vi "Exercise9.2-Basic Sine RX.vi"() -> ()   [LabVIEW 2013]
uses:
  <instrlib>/niUSRP/niUSRP Fetch Rx Data (CDB WDT).vi
  <vilib>/express/express analysis/Spectral/Block/exnSpectralBlock spectral measurements RMS poly.vi
  <vilib>/express/express analysis/Spectral/Block/exnSpectralBlock spectral measurements RMS WFM.vi
  <vilib>/express/express analysis/Spectral/XNode/ExpressSpectralMeasurementsBlockNode.xnode
panel:
  out "Spectrum":cluster{"f0":dbl, "df":dbl, "magnitude":dbl[]}(graph)={"f0"=0.0, "df"=2.0, "magnitude"=array[50000 elements]}
  out "error out":errorcluster
  out "coerced gain":dbl format="%#_6f"
  out "coerced IQ rate":dbl=200000.0 format="%#_6p"
  out "coerced carrier frequency":dbl=2400000000.0 format="%#_6p"
  out "Waveform":waveform(dbl)[](graph)=[{"t0"=timestamp(3637211128.6485267 s since 1904-01-01), "dt"=5e-06, "Y"=array[100000 elements]}, {"t0"=timestamp(3637211128.6485267 s since 1904-01-01), "dt"=5e-06, "Y"=array[100000 elements]}]
  in  "number of samples":i64=100000
  in  "stop":bool
  in  "device names":refnum<k15>="192.168.10.2"
  in  "active antenna":string="RX2"
  in  "gain":dbl format="%#_6f"
  in  "carrier frequency":dbl=2400000000.0 format="%#_6p"
  in  "IQ rate":dbl=200000.0 format="%#_6p"
  # "USRP Receiver"
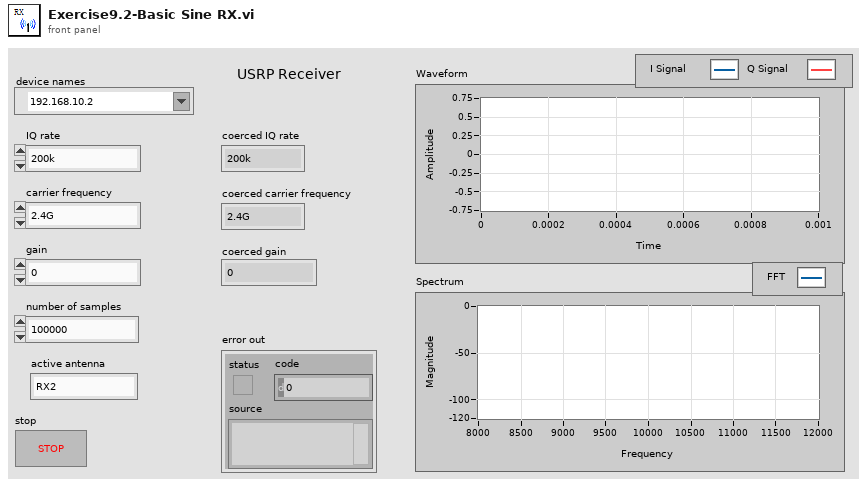
[diagram p1: front panel]
types:
  T1 = cluster{"averaging mode":u16, "weighting mode":u16, "number of averages":u32}
  T2 = cluster{"dB On (F)":bool, "unwrap phase (F)":bool, "convert to degree (F)":bool}
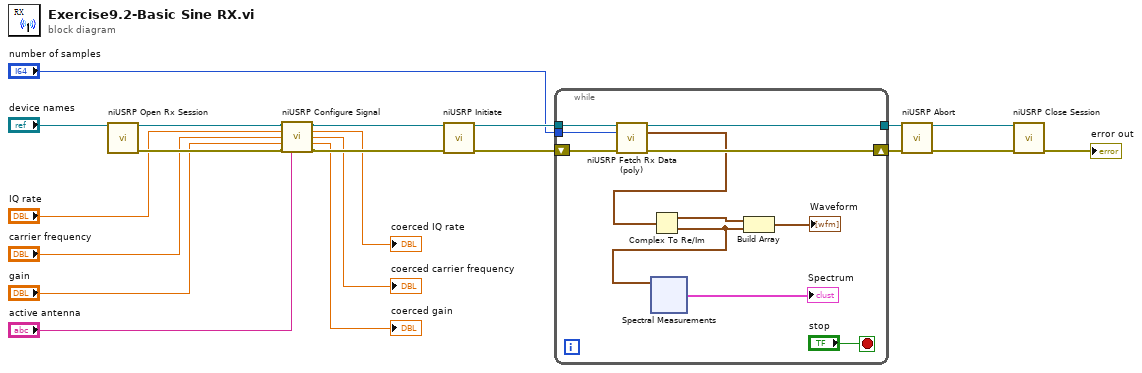
[diagram p0: block diagram]
diagram:
  n1 = call <instrlib>:"niUSRP Open Rx Session.vi"("device names"="device names") -> ("session handle out"=w11:refnum<k15>, "error out"=w12:errorcluster)  [unwired: 13 in]
  n2 = call <instrlib>:"niUSRP Configure Signal.vi"("session handle"=w11, "IQ rate"="IQ rate", "carrier frequency"="carrier frequency", "gain"="gain", "error in (no error)"=w12, "active antenna"="active antenna") -> ("session handle out"=w14:refnum<k15>, "coerced IQ rate"=→"coerced IQ rate":dbl, "coerced carrier frequency"=→"coerced carrier frequency":dbl, "coerced gain"=→"coerced gain":dbl, "error out"=w13:errorcluster)  [unwired: 5 in]
  n3 = call <instrlib>:"niUSRP Initiate.vi"("session handle"=w14, "error in (no error)"=w13) -> ("session handle out"=w20:refnum<k15>, "error out"=w15:errorcluster)  [unwired: 12 in]
  n4 = while {
    shift-right: [w27] -> w16
    shift-left: w15 -> [w28]
    tunnel: w20 -> [w31]
    tunnel: [w30] -> w19
    tunnel: "number of samples" -> [w26]
    stop <- "stop" stop-if-true
    n5 = call-poly <instrlib>:"niUSRP Fetch Rx Data (poly).vi"("session handle"=w31, "number of samples"=w26, "error in (no error)"=w28) -> ("session handle out"=w30:refnum<k15>, "data"=w25:waveform(cdb), "error out"=w27:errorcluster)  [unwired: 9 in, 1 out]
    n6 = Complex To Re/Im(x + iy=w25) -> (x=w24:waveform(dbl), y=w22:waveform(dbl))
    n7 = xnode "Spectral Measurements"("Signals"=w22) -> ("FFT - (RMS)"=→"Spectrum":cluster{"f0":dbl, "df":dbl, "magnitude":dbl[]})  [unwired: 1 in, 2 out]
    n8 = Build Array(w24, w22) -> (→"Waveform":waveform(dbl)[])
  }
  n9 = call <instrlib>:"niUSRP Abort.vi"("session handle"=w19, "error in (no error)"=w16) -> ("session handle out"=w18:refnum<k15>, "error out"=w17:errorcluster)  [unwired: 12 in]
  n10 = call <instrlib>:"niUSRP Close Session.vi"("session handle"=w18, "error in (no error)"=w17) -> ("error out"=→"error out":errorcluster)  [unwired: 13 in]
